vi "Update Button Text.vi"(11 "Buttons":refnum<vi>) -> ()   [LabVIEW 2015, in "UIStep.lvclass"]
uses:
  UIStep.lvclass
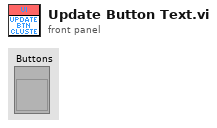
[diagram p1: front panel]
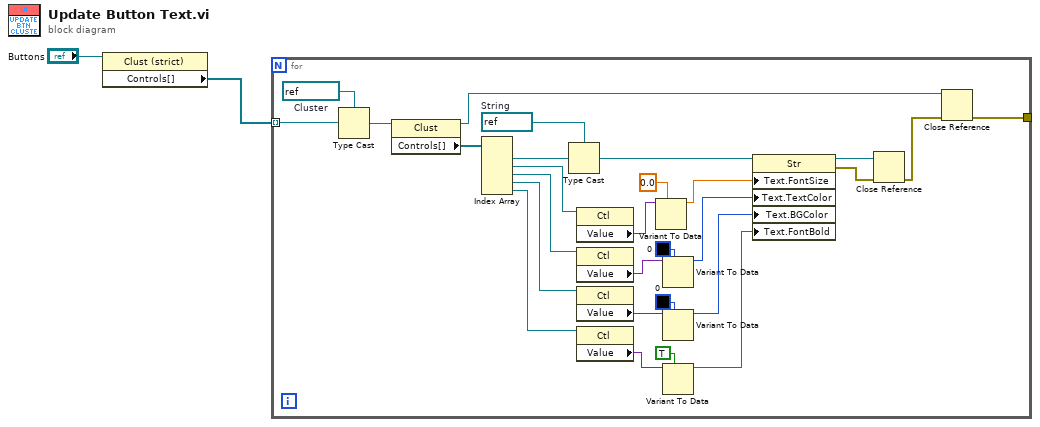
[diagram p0: block diagram]
diagram:
  n1 = property class="Clust (strict)"(reference="Buttons") -> ("Controls[]"=w1:refnum<vi>[])  [unwired: 1 in, 2 out]
  n2 = for {
    tunnel: w1 -> [w30] mode=indexing
    tunnel: [w3] -> _
    w25 = refnum<vi> refnum  # String
    w29 = refnum<vi> refnum  # Cluster
    n3 = Type Cast(type=w29, x=w30) -> (*(type *) &x=w28:refnum<vi>)
    n4 = property class="Clust"(reference=w28) -> (reference out=w6:refnum<vi>, "Controls[]"=w27:refnum<vi>[])  [unwired: 1 in, 1 out]
    n5 = Index Array(array=w27) -> (element #1=w26:refnum<vi>, element #2=w23:refnum<vi>, element #3=w22:refnum<vi>, element #4=w21:refnum<vi>, element #5=w20:refnum<vi>)  [unwired: 5 in]
    n6 = Type Cast(type=w25, x=w26) -> (*(type *) &x=w24:refnum<vi>)
    n7 = property class="Ctl"(reference=w23) -> ("Value"=w10:variant)  [unwired: 1 in, 2 out]
    n8 = property class="Ctl"(reference=w22) -> ("Value"=w12:variant)  [unwired: 1 in, 2 out]
    n9 = property class="Ctl"(reference=w21) -> ("Value"=w16:variant)  [unwired: 1 in, 2 out]
    n10 = property class="Ctl"(reference=w20) -> ("Value"=w19:variant)  [unwired: 1 in, 2 out]
    n11 = Variant To Data(type=0.0, Variant=w10) -> (data=w8:dbl)  [unwired: 1 in, 1 out]
    n12 = Variant To Data(type=u32 0, Variant=w12) -> (data=w11:u32)  [unwired: 1 in, 1 out]
    n13 = Variant To Data(type=u32 0, Variant=w16) -> (data=w14:u32)  [unwired: 1 in, 1 out]
    n14 = Variant To Data(type=TRUE, Variant=w19) -> (data=w17:bool)  [unwired: 1 in, 1 out]
    n15 = property class="Str"(reference=w24, "Text.FontSize"=w8, "Text.TextColor"=w11, "Text.BGColor"=w14, "Text.FontBold"=w17) -> (reference out=w7:refnum<vi>, error out=w4:errorcluster)  [unwired: 1 in]
    n16 = Close Reference(reference=w7, error in (no error)=w4) -> (error out=w5:errorcluster)
    n17 = Close Reference(reference=w6, error in (no error)=w5) -> (error out=w3:errorcluster)
  }
